vi "Find_calibration_file.vi"(1 "Inst type":T1=enum."Pressure Transducer", 2 "Channel ID":string, 3 "Use Latest Calib":bool, 4 "filename":path) -> (0 "filename out":path)   [LabVIEW 2022 SP3]
uses:
  Controls/Inst_type.ctl
  Controls/App_Global.ctl
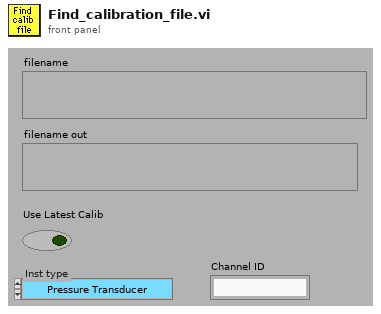
[diagram p1: front panel]
types:
  T1 = typedef "Inst_type.ctl" = enum16{"Raw voltage", "Raw with zero offsetting", "Propeller anemometer", "Pressure Transducer", "Pitot-static tube", "Hot wire", "Cross wire 1", "Cross wire 2", "Generic Linear", "Generic Polynomial", "Generic BackPoly", "Fast FID", "Thermocouple", "Cold wire", "Pulsed Wire", "LDA Vel", "LDA Tran time", "LDA Arr time", "Microphone"}
  T2 = typedef "App_Global.ctl" = enum16{"Read Global", "Write to Global", "Initialise Array"}
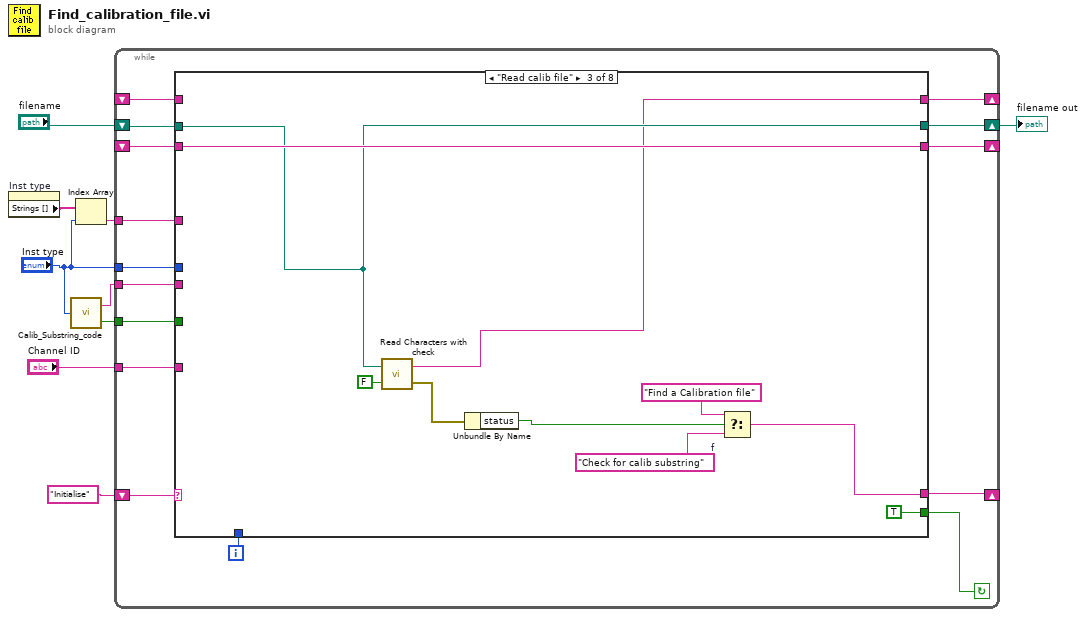
[diagram p0: block diagram]
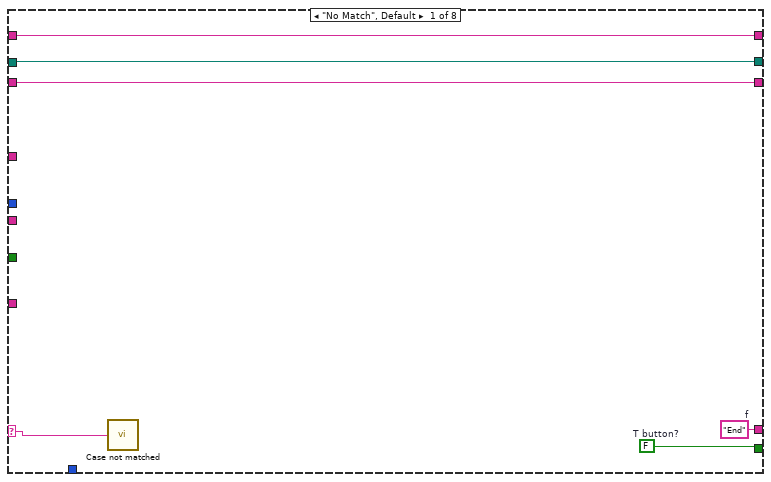
[diagram p2: hidden frame]
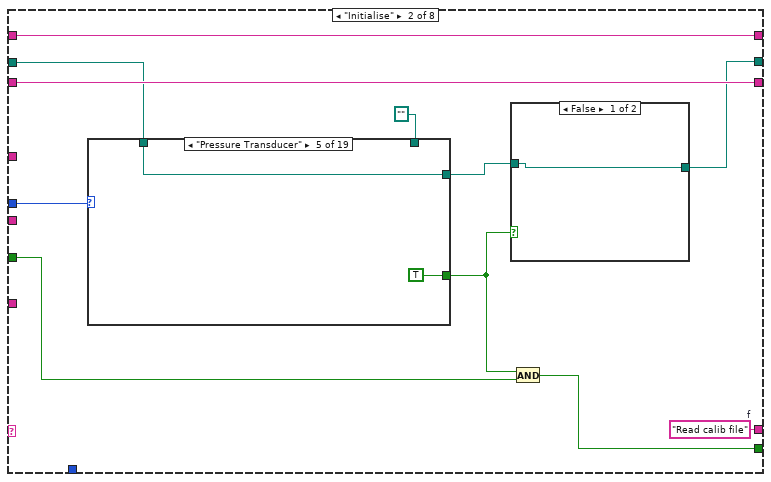
[diagram p3: hidden frame]
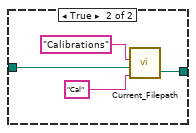
[diagram p4: hidden frame]
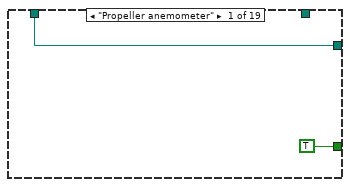
[diagram p5: hidden frame]
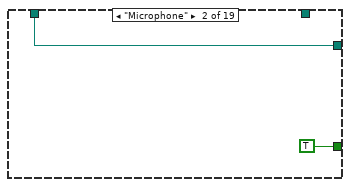
[diagram p6: hidden frame]
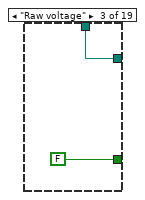
[diagram p7: hidden frame]
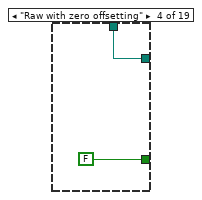
[diagram p8: hidden frame]
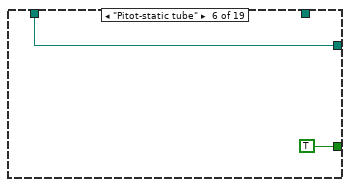
[diagram p9: hidden frame]
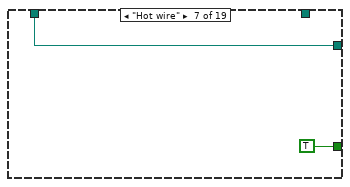
[diagram p10: hidden frame]
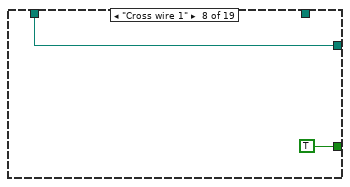
[diagram p11: hidden frame]
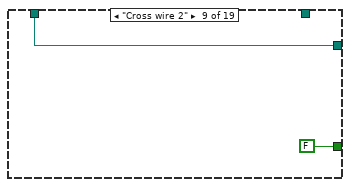
[diagram p12: hidden frame]
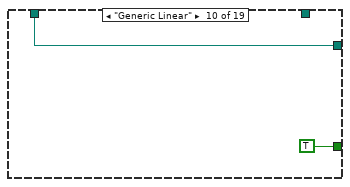
[diagram p13: hidden frame]
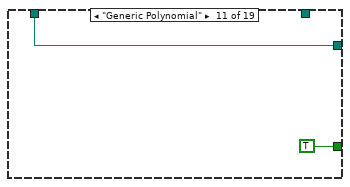
[diagram p14: hidden frame]
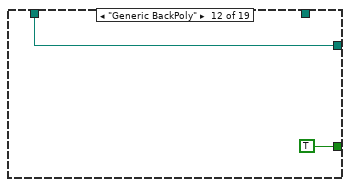
[diagram p15: hidden frame]
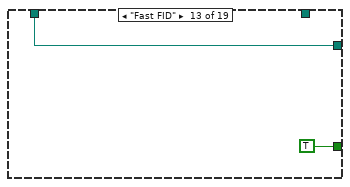
[diagram p16: hidden frame]
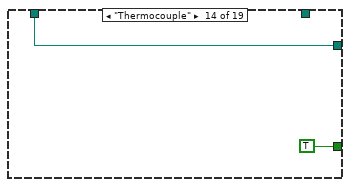
[diagram p17: hidden frame]
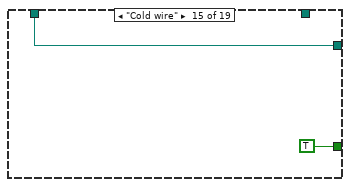
[diagram p18: hidden frame]
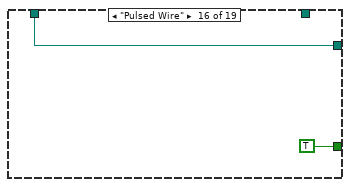
[diagram p19: hidden frame]
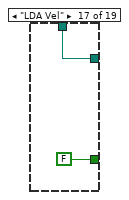
[diagram p20: hidden frame]
diagram:
  n1 = property on="Inst type" class="Enum (strict)"() -> ("Strings []"=w6:string[])  [unwired: 2 in, 2 out]
  n2 = call "Calib_Substring_code.vi"("Inst type"="Inst type") -> ("Substring Type"=w3:string, "Read file"=w2:bool)
  n3 = Index Array(array=w6, index="Inst type") -> (element=w5:string)
  n4 = while {
    shift-left: "filename" -> [w24]
    shift-right: [w23] -> w8
    shift-left: "Initialise" -> [w17]
    shift-right: [w22] -> _
    shift-right: [w19] -> _
    shift-left: _ -> [w18]
    tunnel: "Inst type" -> [w16]
    tunnel: w5 -> [w15]
    shift-right: [w13] -> _
    shift-left: _ -> [w14]
    tunnel: w3 -> [w12]
    tunnel: w2 -> [w11]
    tunnel: "Channel ID" -> [w10]
    i -> [w20]
    stop <- w21 continue-if-true
    n5 = case shown="\"Read calib file\"" w17 {
      tunnel: w24 -> [w29 w37 w88 w100 w110 w137 w168 w197]
      selector: w17 -> [w25 _ _ _ _ _ _ _]
      tunnel: [w29 w32 w88 w97 w110 w137 w168 w197] -> w23
      tunnel: [w28 w38 w92 "Update Lastest Calib?" w115 w146 "Find a Calibration file" "Read calib file" ("f")] -> w22
      tunnel: [w27 w34 TRUE w106 w118 w147 w183 w195] -> w21
      tunnel: w20 -> [_ _ _ _ _ _ _ _]
      tunnel: [w30 w41 w87 w108 w113 w144 w170 w199] -> w19
      tunnel: w18 -> [w30 w41 _ w108 w113 w144 w170 w199]
      tunnel: w16 -> [_ w39 _ _ _ w145 _ _]
      tunnel: w15 -> [_ _ _ w104 w116 _ _ _]
      tunnel: w14 -> [w26 w40 w90 w105 _ w135 w171 w198]
      tunnel: [w26 w40 w90 w105 w114 w135 w171 w198] -> w13
      tunnel: w12 -> [_ _ _ _ w112 _ _ _]
      tunnel: w11 -> [_ w35 _ _ _ _ _ _]
      tunnel: w10 -> [_ _ _ w102 _ _ _ w194]
      frame "No Match", Default {
        w27 = FALSE  # T button?
        w28 = "End"  # f
        n6 = call "Case not matched.vi"("Case Name not Matched"=w25) -> ()
      }
      frame "Initialise" {
        w38 = "Read calib file"  # f
        n7 = case shown="\"Pressure Transducer\"" w39 {
          tunnel: [TRUE TRUE FALSE FALSE TRUE TRUE TRUE TRUE FALSE TRUE TRUE TRUE TRUE TRUE TRUE TRUE FALSE FALSE FALSE] -> w31
          tunnel: [w47 w49 w51 w53 w55 w57 w59 w61 w63 w65 w67 w69 w71 w73 w75 w77 w79 w81 w83] -> w33
          tunnel: w37 -> [w47 w49 _ _ w55 w57 w59 w61 w63 w65 w67 w69 w71 w73 w75 w77 _ _ _]
          tunnel: path "" -> [_ _ w51 w53 _ _ _ _ _ _ _ _ _ _ _ _ w79 w81 w83]
          frame "Propeller anemometer" {
          }
          frame "Microphone" {
          }
          frame "Raw voltage" {
          }
          frame "Raw with zero offsetting" {
          }
          frame "Pressure Transducer" {
          }
          frame "Pitot-static tube" {
          }
          frame "Hot wire" {
          }
          frame "Cross wire 1" {
          }
          frame "Cross wire 2" {
          }
          frame "Generic Linear" {
          }
          frame "Generic Polynomial" {
          }
          frame "Generic BackPoly" {
          }
          frame "Fast FID" {
          }
          frame "Thermocouple" {
          }
          frame "Cold wire" {
          }
          frame "Pulsed Wire" {
          }
          frame "LDA Vel" {
          }
          frame "LDA Tran time" {
          }
          frame "LDA Arr time" {
          }
        }
        n8 = case shown="False" w31 {
          tunnel: w33 -> [w42 w44]
          tunnel: [w42 w43] -> w32
          frame False {
          }
          frame True {
            n9 = call "Current_Filepath.vi"("Short_Name"="Cal" ("Data Type"), "Filename in"=w44, "Data Type"="Calibrations") -> ("Filename Out"=w43:path)  [unwired: 1 in, 1 out]
          }
        }
        n10 = And(x=w31, y=w35) -> (x .and. y?=w34:bool)
      }
      frame "Read calib file" {
        w91 = "Check for calib substring"  # f
        n11 = call "Read Characters with check.vi"("Call EnFlo Error Handler?"=FALSE, "file (use dialog)"=w88) -> ("error out"=w86:errorcluster, "Read String"=w87:string)
        n12 = Unbundle By Name(w86) -> ("status"=w89:bool)
        n13 = Select(t="Find a Calibration file", s=w89, f=w91) -> (s? t:f=w92:string)
      }
      frame "Find a Calibration file" {
        n14 = Format Into String(format string=" calibration file for channel %s not found.  Please search for it.", initial string=w104, w102) -> (resulting string=w96:string)  [unwired: 1 in, 1 out]
        n15 = call "Current_Filepath.vi"("Short_Name"="Cal" ("Data Type"), "Filename in"=w100, "Data Type"="Calibrations") -> ("Directory"=w99:path)  [unwired: 1 in, 1 out]
        n16 = call "File Dialog"("start path"=w99, "prompt"=w96) -> ("selected path"=w97:path, "cancelled"=w98:bool)  [unwired: 10 in, 2 out]
        n17 = Not(x=w98) -> (.not. x?=w106:bool)
      }
      frame "Check for calib substring" {
        w120 = FALSE  # Show Dialog?
        n18 = Concatenate Strings(w112, "calib label") -> (w117:string)
        n19 = Format Into String(format string="Calibration File   %s", w110) -> (resulting string=w109:string)  [unwired: 2 in, 1 out]
        n20 = call "Get_string_subset.vi"("String Name"=w109, "Show Dialog?"=w120, "String to split"=w113, "File Label"=w117) -> ("Status"=w119:enum16{"Char in string", "Char not in string"}, "Output string"=w114:string)
        n21 = case shown="\"Char in string\"" w119 {
          tunnel: [TRUE w129] -> w118
          tunnel: w110 -> [_ w125]
          tunnel: w116 -> [_ w128]
          tunnel: ["Was there sufficient calibration points?" "Find a Calibration file"] -> w115
          frame "Char in string" {
          }
          frame "Char not in string" {
            w126 = "The calibration file\n\"%s\"\nis not the appropriate file for a %s"  # format string
            w130 = "Find another file"  # T button name ("OK")
            n22 = Strip Path(path=w125) -> (name=w124:string)  [unwired: 1 out]
            n23 = Format Into String(format string=w126, w124, w128) -> (resulting string=w131:string)  [unwired: 2 in, 1 out]
            n24 = Two Button Dialog(message=w131, 2:w130) -> (T button?=w129:bool)  [unwired: 1 out]
          }
        }
      }
      frame "Was there sufficient calibration points?" {
        n25 = Format Into String(format string="Calibration File   %s", w137) -> (resulting string=w134:string)  [unwired: 2 in, 1 out]
        n26 = call "2D_String_array_from_string.vi"("String Name"=w134, "Input string"=w135, "Array title"="Calib points label") -> ("2D data array"=w133:string[][])
        n27 = for {
          tunnel: w133 -> [w154] mode=indexing
          tunnel: [w148] -> w140 mode=indexing
          tunnel: "NaN" -> [w149]
          n28 = Index Array(array=w154, index=5) -> (element=w152:string)
          n29 = String Subset(string=w152, length (rest)=3 ("length (rest)")) -> (substring=w150:string)  [unwired: 1 in]
          n30 = Not Equal?(x=w149, y=w150) -> (x != y?=w148:bool)
        }
        n31 = Boolean To (0,1)(Boolean=w140) -> (0, 1=w143:i16[])
        n32 = Add Array Elements(numeric array=w143) -> (sum=w141:i16)
        n33 = Greater?(x=w141, y=i16 1) -> (0:w139:bool)
        n34 = case shown="False" w139 {
          tunnel: [w159 w163] -> w147
          tunnel: w137 -> [w156 _]
          tunnel: ["Find a Calibration file" "Are XW psi 1 and 2 valid"] -> w146
          tunnel: w145 -> [_ w164]
          frame False {
            w157 = "The calibration file\n\"%s\"\nhas less than two calibration points."  # format string
            w160 = "Find another file"  # T button name ("OK")
            n35 = Strip Path(path=w156) -> (name=w155:string)  [unwired: 1 out]
            n36 = Format Into String(format string=w157, w155) -> (resulting string=w161:string)  [unwired: 2 in, 1 out]
            n37 = Two Button Dialog(message=w161, 2:w160) -> (T button?=w159:bool)  [unwired: 1 out]
          }
          frame True {
            n38 = case shown="\"Propeller anemometer\", Default" w164 {
              tunnel: [FALSE TRUE] -> w163
              frame "Propeller anemometer", Default {
              }
              frame "Cross wire 1" {
              }
            }
          }
        }
      }
      frame "Are XW psi 1 and 2 valid" {
        w176 = FALSE  # Show Dialog?
        n39 = Build Array("C0", "C1", "C2") -> (w178:string[])
        n40 = Format Into String(format string="Calibration File   %s", w168) -> (resulting string=w167:string)  [unwired: 2 in, 1 out]
        n41 = call "Get_string_subset.vi"("String Name"=w167, "Show Dialog?"=w176, "String to split"=w170, "File Label"="Auxiliary constants") -> ("Output string"=w177:string)  [unwired: 1 out]
        n42 = for {
          tunnel: w178 -> [w186] mode=indexing
          tunnel: [w185] -> w175 mode=indexing
          tunnel: w177 -> [w184]
          n43 = call "Get_value_from_string.vi"("Input string"=w184, "Variable name"=w186) -> ("Value"=w185:dbl)  [unwired: 1 in, 1 out]
        }
        n44 = Not A Number/Path/Refnum?(number/path/refnum=w175) -> (NaN/Path/Refnum?=w174:bool[])
        n45 = Or Array Elements(Boolean array=w174) -> (logical OR=w173:bool)
        n46 = case shown="False" w173 {
          tunnel: [FALSE w191] -> w183
          tunnel: w168 -> [_ w189]
          frame False {
          }
          frame True {
            n47 = Strip Path(path=w189) -> (name=w188:string)  [unwired: 1 out]
            n48 = Format Into String(format string="The XW calibration file\n\"%s\"\ndoes not have valid angle calibration coefficients.", w188) -> (resulting string=w193:string)  [unwired: 2 in, 1 out]
            n49 = Two Button Dialog(message=w193, 2:"Find another file" ("T button name (\"OK\")")) -> (T button?=w191:bool)  [unwired: 1 out]
          }
        }
      }
      frame "Update Lastest Calib?" {
        w195 = TRUE  # T button?
        n50 = case shown="True" "Use Latest Calib" {
          tunnel: w197 -> [_ w204]
          tunnel: w194 -> [_ w201]
          frame False {
          }
          frame True {
            n51 = Build Array(w204) -> (w202:path[])
            n52 = Build Array(w201) -> (w203:string[])
            n53 = call "Current_Calib_Filenames.vi"("Calib Filename"=w202, "Channel ID input"=w203, "Mode"=App_Global."Write to Global") -> ()  [unwired: 3 out]
          }
        }
      }
    }
  }
  "filename out" <- w8
